vi "cyclical_counter.vi"(1 "Enable":bool, 2 "Mod":u16) -> (0 "Count":u16)   [LabVIEW 2018]
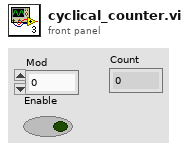
[diagram p1: front panel]
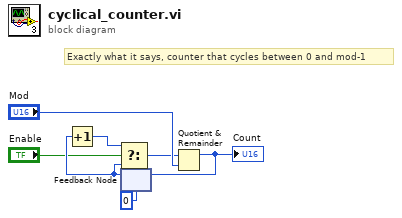
[diagram p0: block diagram]
diagram:
  # "Exactly what it says, counter that cycles between 0 and mod-1"
  n1 = feedback #1(u16 0) -> (w6:u16)
  n2 = Increment(x=w6) -> (x+1=w7:u16)
  n3 = Select(t=w7, s="Enable", f=w6) -> (s? t:f=w2:u16)
  n4 = Quotient & Remainder(x=w2, y="Mod") -> (x-y*floor(x/y)=w1:u16)  [unwired: 1 out]
  "Count" <- w1
  n5 = feedback-in #1(w1) -> ()
